vi "configuration_read.vi"(8 "error in (no error)":errorcluster, 11 "lv-build in":refnum<class "lv-builder-default.lvclass">) -> (0 "error out":errorcluster, 2 "configuration":variant, 3 "lv-build out":refnum<class "lv-builder-default.lvclass">)   [LabVIEW 2015, in "lv-builder-default.lvclass"]
uses:
  lv-builder-default.lvclass
  lv-builder-default.lvclass/lv-builder-default.ctl
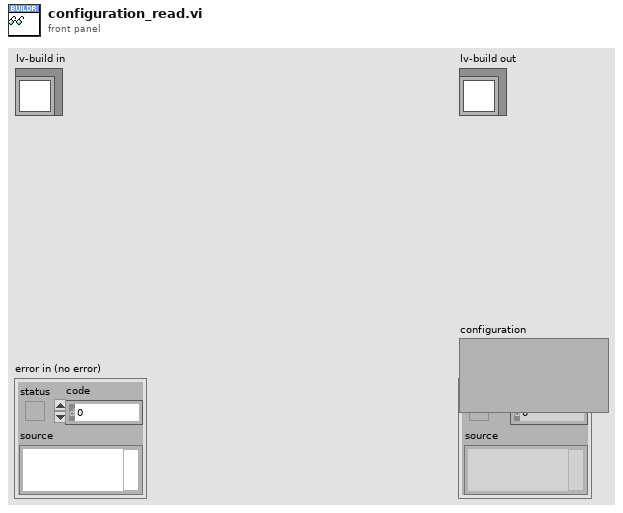
[diagram p1: front panel]
types:
  T1 = typedef "lv-builder-default.lvlib/configuration.ctl" = cluster{"project_file":string, "lvlibp_directory":string, "zip_directory":string, "lvlib_directory":string, "update_version_vi":string, "installer_post_file":string, "distribution_folder":string, "dependencies_folder":string, "version":string, "bin_folder":string, "lvlib_post_action":u16, "installer_post_action":u16, "application_post_action":u16, "zip_post_action":u16}
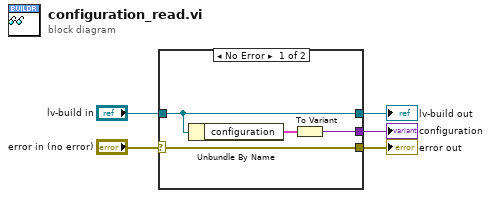
[diagram p0: block diagram]
diagram:
  n1 = case shown="No Error" "error in (no error)" {
    selector: "error in (no error)" -> [w9 w10]
    tunnel: [w9 w10] -> w5
    tunnel: [w7 _] -> w4
    tunnel: "lv-build in" -> [w6 w11]
    tunnel: [w6 w11] -> w1
    frame No Error {
      n2 = Unbundle By Name(w6) -> ("configuration"=w8:T1)
      n3 = To Variant(anything=w8) -> (Variant=w7:variant)
    }
    frame Error {
    }
  }
  "error out" <- w5
  "lv-build out" <- w1
  "configuration" <- w4
